vi "Set Variables.vi"(8 "error in (no error)":errorcluster, 10 "Variables":variant, 11 "functionbase in":refnum<class "functionbase.lvclass">) -> (0 "error out":errorcluster, 3 "functionbase out":refnum<class "functionbase.lvclass">)   [LabVIEW 2016, in "functionbase.lvclass"]
uses:
  functionbase.lvclass
  typedefs/Variables.ctl
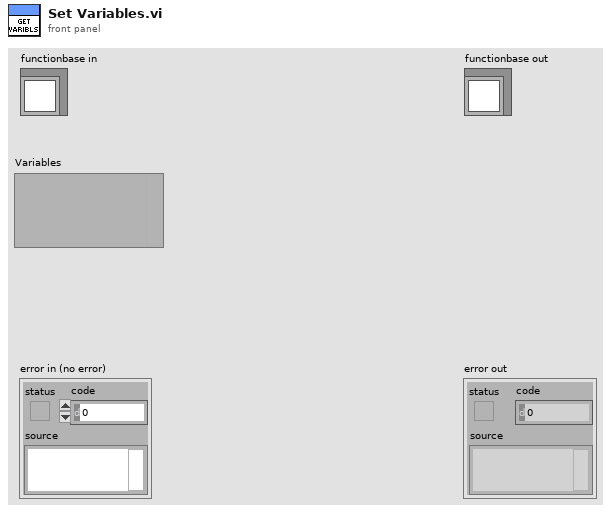
[diagram p1: front panel]
types:
  T1 = typedef "functionbase.lvclass/Variables.ctl" = cluster{"BoringEngineer":string}
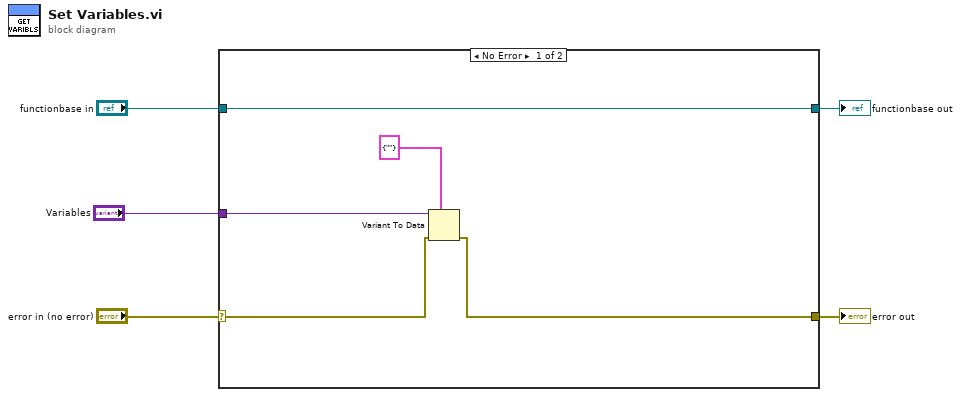
[diagram p0: block diagram]
diagram:
  n1 = case shown="No Error" "error in (no error)" {
    selector: "error in (no error)" -> [w7 w12]
    tunnel: [w6 w12] -> w4
    tunnel: [w10 w11] -> w2
    tunnel: "functionbase in" -> [w10 w11]
    tunnel: "Variables" -> [w9 _]
    frame No Error {
      n2 = Variant To Data(error in=w7, type=T1 {"BoringEngineer"=""} ("Variables"), Variant=w9) -> (error out=w6:errorcluster)  [unwired: 1 out]
    }
    frame Error {
    }
  }
  "error out" <- w4
  "functionbase out" <- w2
